vi "Move test.vi"() -> ()   [LabVIEW 2013]
panel:
  out "Voltage":dbl(graph)
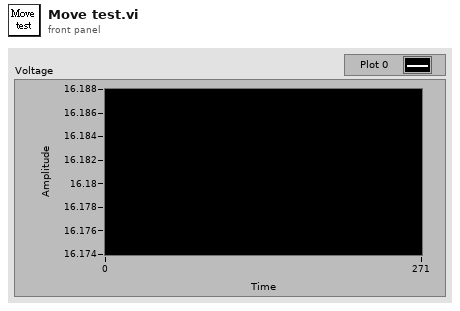
[diagram p1: front panel]
types:
  T1 = typedef "KNR3 Reference.ctl" = cluster{"FPGA Session":refnum<class "FPGA Interface Base.lvclass">, "Resource":T2}
  T2 = typedef "Resource.ctl" = enum16{"KNRm_DDRC", "KNRm_DDDD", "KNRm_DDDR", "KNRm_DDDC", "KNR"}
  T3 = cluster{"Mode":enum16{"FRWD", "TURFIX", "TURNOF", "CIRCULAR"}, "Dir":enum16{"Left", "Right"}, "Pcmd":dbl, "Vcmd":dbl, "X":dbl, "Y":dbl}
  T4 = cluster{"Mode":enum16{"FRWD", "TURFIX", "TURNOF"}, "Dir":enum16{"Left", "Right"}, "Pcmd":dbl, "Vcmd":dbl}
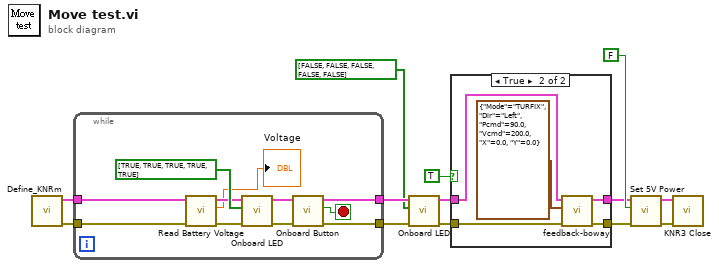
[diagram p0: block diagram]
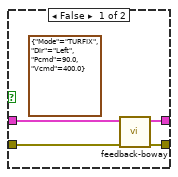
[diagram p2: hidden frame]
diagram:
  n1 = call "Define_KNRm.vi"() -> ("error out"=w13:errorcluster, "KNR out"=w12:T1)  [unwired: 10 in]
  n2 = while {
    tunnel: [w23] -> w11
    tunnel: [w21] -> w9
    tunnel: w12 -> [w16]
    tunnel: w13 -> [w15]
    stop <- w24 stop-if-true
    n3 = call <userlib>:"Read Battery Voltage.vi"("error in (no error)"=w15, "KNR in"=w16) -> ("error out"=w17:errorcluster, "Voltage"=→"Voltage":dbl, "KNR out"=w18:T1)  [unwired: 7 in]
    n4 = call <userlib>:"Onboard LED.vi"("error in (no error)"=w17, "LED List"=bool[] [TRUE, TRUE, TRUE, TRUE, TRUE], "KNR in"=w18) -> ("error out"=w22:errorcluster, "KNR out"=w20:T1)  [unwired: 7 in]
    n5 = call <userlib>:"Onboard Button.vi"("error in (no error)"=w22, "KNR in"=w20) -> ("error out"=w21:errorcluster, "value"=w24:bool, "KNR out"=w23:T1)  [unwired: 7 in]
  }
  n6 = call <userlib>:"Onboard LED.vi"("error in (no error)"=w9, "LED List"=bool[] [FALSE, FALSE, FALSE, FALSE, FALSE], "KNR in"=w11) -> ("error out"=w1:errorcluster, "KNR out"=w2:T1)  [unwired: 7 in]
  n7 = case shown="True" TRUE {
    tunnel: w1 -> [w28 w32]
    tunnel: [w27 w31] -> w5
    tunnel: w2 -> [w26 w33]
    tunnel: [w25 w30] -> w4
    frame False {
      (unwired) T4 {"Mode"=enum."TURFIX", "Dir"=enum."Left", "Pcmd"=90.0, "Vcmd"=400.0} ("Move")
      n8 = call "feedback-boway.vi"("error in (no error)"=w28, "KNR in"=w26) -> ("error out"=w27:errorcluster, "KNR out"=w25:T1)  [unwired: 7 in, 1 out]
    }
    frame True {
      n9 = call "feedback-boway.vi"("error in (no error)"=w32, "Move"=T3 {"Mode"=enum."TURFIX", "Dir"=enum."Left", "Pcmd"=90.0, "Vcmd"=200.0, "X"=0.0, "Y"=0.0}, "KNR in"=w33) -> ("error out"=w31:errorcluster, "KNR out"=w30:T1)  [unwired: 6 in, 1 out]
    }
  }
  n10 = call <userlib>:"Set 5V Power.vi"("error in (no error)"=w5, "5V Power(T)"=FALSE, "KNR in"=w4) -> ("error out"=w8:errorcluster, "KNR out"=w7:T1)  [unwired: 7 in]
  n11 = call <userlib>:"KNR3 Close.vi"("error in (no error)"=w8, "KNR in"=w7) -> ()  [unwired: 9 in, 1 out]
